vi "_Save All Tables.vi"(4 "error in (no error)":errorcluster, 5 "FilePath(My Table.tbl)":string="My Tables.tbl", 7 "SaveOption (Temporary File)":T1=enum."Temporary File") -> (0 "error out":errorcluster, 1 "Path":path)   [LabVIEW 2015]
uses:
  Type/_SaveOption.ctl
  Type/_RT Command.ctl
  Type/_RT Configuration 2.ctl
  <vilib>/Utility/config.llb/Read Key (String).vi
  Configuration/_Global Configuration.vi
  <vilib>/Utility/config.llb/NI_LVConfig.lvlib
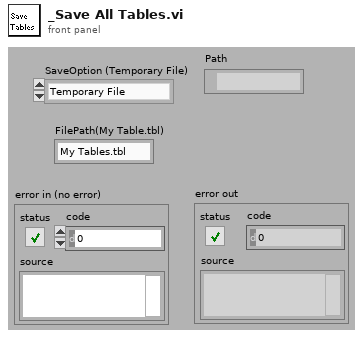
[diagram p1: front panel]
types:
  T1 = typedef "_SaveOption.ctl" = enum16{"Use Dialog", "Temporary File", "My Tables", "Full Path"}
  T2 = typedef "_RT Configuration 2.ctl" = cluster{"Name":string, "Ch#":u8, "Min":dbl, "Max":dbl, "Def+":dbl, "Def-":dbl, "Offset":dbl, "Slope":dbl, "Type":u8, "Description":string, "SettleT":dbl}
  T3 = typedef "_RT Command.ctl" = enum16{"Start", "StartActualRun", "Stop", "Runtime Update", "Get Data", "Get Info", "Get Status", "Get Param", "Get Config", "Get Table", "Read ADC", "Set Oscillator", "Update Config", "Update Table", "Set All Pol", "Set Pol and DC", "Set Max Mass", "Toggle RP", "Toggle EL", "Set PIC", "Initialize Turbo", "Send Turbo Comm", "Close Turbo", "P1", "P2", "P3", "Send Serial", "Set LC Out", "Get LC In", "Read VAC", "Test Table", "Toggle Power", "Get Startup", "Set Startup", "Get ADC Table", "Set ADC Table", "Get Brief Status", "Get Detail Status", "Auxiliary Update", "Set CC Logics", "Set CC Input Logics", "Ignore Error"}
  T4 = enum32{"existing file", "new file", "new or existing file", "existing dir", "new dir", "new or existing dir", "existing file (use LLBs)", "new file (use LLBs)", "new or existing file (use LLBs)", "new or existing file or directory (use LLBs)"}
  T5 = typedef "NI_LVConfig.lvlib/Config Data RefNum.ctl" = refnum<k1>
  T6 = enum16{"open", "replace", "create", "open or create", "replace or create", "replace or create with confirmation"}
  T7 = typedef "_RT Instrument 2.ctl" = cluster{"Table":T2[], "Instrument":string[]}
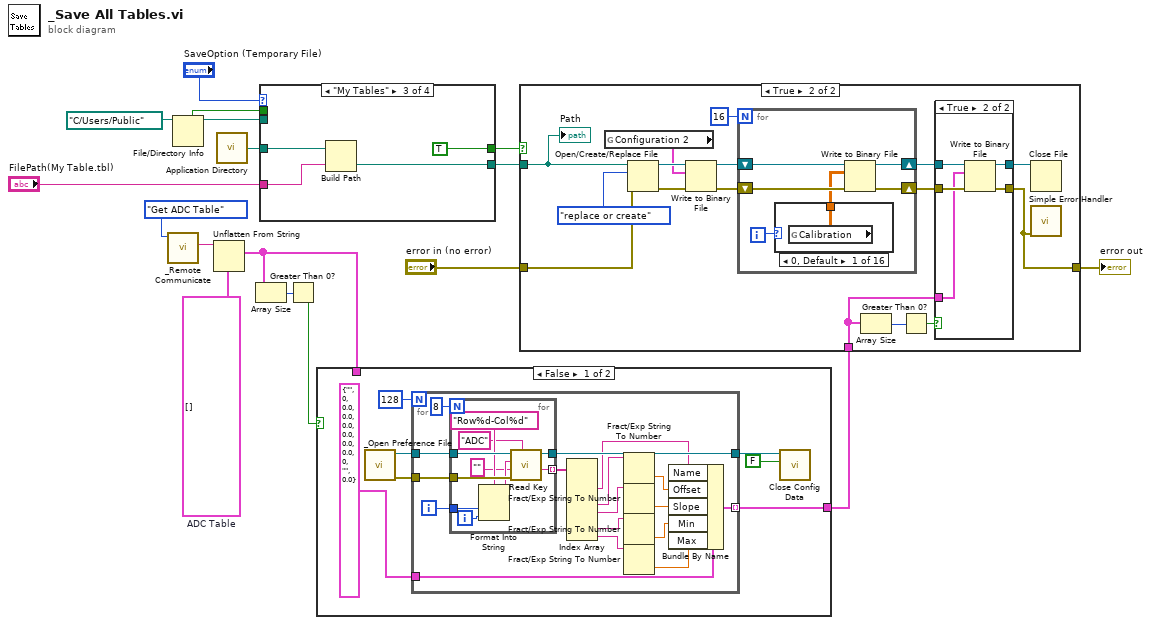
[diagram p0: block diagram]
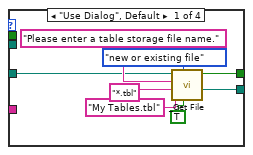
[diagram p3: hidden frame]
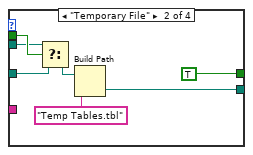
[diagram p4: hidden frame]
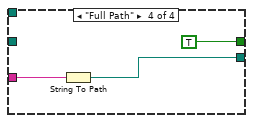
[diagram p5: hidden frame]
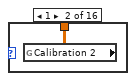
[diagram p8: hidden frame]
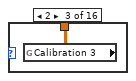
[diagram p9: hidden frame]
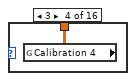
[diagram p10: hidden frame]
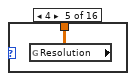
[diagram p11: hidden frame]
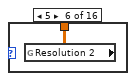
[diagram p12: hidden frame]
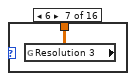
[diagram p13: hidden frame]
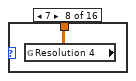
[diagram p14: hidden frame]
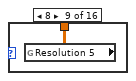
[diagram p15: hidden frame]
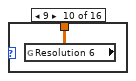
[diagram p16: hidden frame]
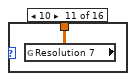
[diagram p17: hidden frame]
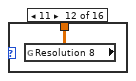
[diagram p18: hidden frame]
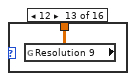
[diagram p19: hidden frame]
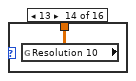
[diagram p20: hidden frame]
diagram:
  w11 = T2[] []  # ADC Table
  n1 = call "_Remote Communicate.vi"("Command"=_RT_Command."Get ADC Table") -> ("Info"=w13:string)  [unwired: 5 in, 3 out]
  n2 = File/Directory Info(path=path "C:/Users/Public" ("stripped path")) -> (path out=w5:path, directory=w6:bool)  [unwired: 1 in, 5 out]
  n3 = Unflatten From String(type=w11, binary string=w13) -> (value=w9:T2[])  [unwired: 1 in, 4 out]
  n4 = call <vilib>:"Application Directory.vi"() -> ("Application Directory"=w1:path)
  n5 = Array Size(array=w9) -> (size(s)=w14:i32)
  n6 = case shown="\"My Tables\"" "SaveOption (Temporary File)" {
    tunnel: w1 -> [w21 w28 w36 _]
    tunnel: [w20 w31 w35 w37] -> w17
    tunnel: [w18 TRUE TRUE TRUE] -> w16
    tunnel: w6 -> [_ w29 _ _]
    tunnel: w5 -> [_ w27 _ _]
    tunnel: "FilePath(My Table.tbl)" -> [_ _ w33 w38]
    frame "Use Dialog", Default {
      n7 = call "_Get File.vi"("For Write (T)"=TRUE, "select mode (new or existing)"=T4."new or existing file", "default name"="My Tables.tbl", "extension (isd)"="*.tbl" ("pattern (all files)"), "prompt"="Please enter a table storage file name.", "Start Path"=w21) -> ("Seleted File"=w20:path, "Succeeded"=w18:bool)  [unwired: 2 out]
    }
    frame "Temporary File" {
      n8 = Select(t=w27, s=w29, f=w28) -> (s? t:f=w26:path)
      n9 = Build Path(base path=w26, name or relative path="Temp Tables.tbl") -> (appended path=w31:path)
    }
    frame "My Tables" {
      n10 = Build Path(base path=w36, name or relative path=w33) -> (appended path=w35:path)
    }
    frame "Full Path" {
      n11 = String To Path(string=w38) -> (path=w37:path)
    }
  }
  n12 = Greater Than 0?(x=w14) -> (x > 0?=w10:bool)
  n13 = case shown="False" w10 {
    tunnel: [w40 w74] -> w8
    tunnel: w9 -> [_ w74]
    frame False {
      n14 = call "_Open Preference File.vi"() -> ("error"=w46:errorcluster, "refnum"=w45:T5)  [unwired: 2 in, 4 out]
      n15 = for {
        N: 128 -> [_]
        tunnel: w45 -> [w63]
        tunnel: w46 -> [w62]
        tunnel: [w60] -> w42
        tunnel: T2 {"Name"="", "Ch#"=0, "Min"=0.0, "Max"=0.0, "Def+"=0.0, "Def-"=0.0, "Offset"=0.0, "Slope"=0.0, "Type"=0, "Description"="", "SettleT"=0.0} ("Configuration") -> [w48]
        tunnel: [w47] -> w40 mode=indexing
        i -> [w59]
        n16 = for {
          N: 8 -> [_]
          tunnel: w63 -> [w73]
          tunnel: w62 -> [w72]
          tunnel: [w71] -> w60
          tunnel: w59 -> [w69]
          tunnel: [w66] -> w54 mode=indexing
          i -> [w70]
          n17 = Format Into String(format string="Row%d-Col%d" ("section"), w69, w70) -> (resulting string=w67:string)  [unwired: 2 in, 1 out]
          n18 = call-poly <vilib>:"Read Key.vi"("section"="ADC", "error in (no error)"=w72, "default value"="", "key"=w67, "refnum"=w73) -> ("value"=w66:string, "refnum out"=w71:T5)  [unwired: 1 in, 4 out]
        }
        n19 = Index Array(array=w54) -> (element #2=w53:string, element #4=w55:string, element #5=w56:string, element #7=w57:string, element #8=w58:string)  [unwired: 8 in, 3 out]
        n20 = Fract/Exp String To Number(string=w55) -> (number=w49:dbl)  [unwired: 4 out]
        n21 = Fract/Exp String To Number(string=w56) -> (number=w50:dbl)  [unwired: 4 out]
        n22 = Fract/Exp String To Number(string=w57) -> (number=w51:dbl)  [unwired: 4 out]
        n23 = Fract/Exp String To Number(string=w58) -> (number=w52:dbl)  [unwired: 4 out]
        n24 = Bundle By Name(cluster=w48, "Name"=w53, "Offset"=w49, "Slope"=w50, "Min"=w51, "Max"=w52) -> (w47:T2)
      }
      n25 = call <vilib>:"Close Config Data.vi"("write file if changed (T)"=FALSE ("write configuration file? (T)"), "refnum"=w42) -> ()  [unwired: 1 in, 9 out]
    }
    frame True {
    }
  }
  n26 = case shown="True" w16 {
    tunnel: w17 -> [_ w79]
    tunnel: w8 -> [_ w80]
    tunnel: "error in (no error)" -> [w75 w78]
    tunnel: [w75 w77] -> w3
    frame False {
    }
    frame True {
      n27 = global read "_Global Configuration.vi" "Configuration 2"() -> (w89:T7)
      n28 = Open/Create/Replace File(file path (use dialog)=w79, error in=w78, operation (0:open)=T6."replace or create") -> (refnum out=w91:refnum<file>, error out=w90:errorcluster)  [unwired: 3 in, 1 out]
      n29 = Write to Binary File(file (use dialog)=w91, data=w89, error in=w90) -> (refnum out=w87:refnum<file>, error out=w88:errorcluster)  [unwired: 4 out]
      n30 = for {
        N: 16 -> [_]
        shift-right: [w99] -> w82
        shift-left: w88 -> [w102]
        shift-right: [w100] -> w83
        shift-left: w87 -> [w103]
        i -> [w104]
        n31 = case shown="0, Default" w104 {
          tunnel: [w105 w106 w107 w108 w109 w110 w111 w112 w113 w114 w115 w116 w117 w118 w119 w120] -> w101
          frame 0, Default {
            n32 = global read "_Global Configuration.vi" "Calibration"() -> (w105:dbl[][])
          }
          frame 1 {
            n33 = global read "_Global Configuration.vi" "Calibration 2"() -> (w106:dbl[][])
          }
          frame 2 {
            n34 = global read "_Global Configuration.vi" "Calibration 3"() -> (w107:dbl[][])
          }
          frame 3 {
            n35 = global read "_Global Configuration.vi" "Calibration 4"() -> (w108:dbl[][])
          }
          frame 4 {
            n36 = global read "_Global Configuration.vi" "Resolution"() -> (w109:dbl[][])
          }
          frame 5 {
            n37 = global read "_Global Configuration.vi" "Resolution 2"() -> (w110:dbl[][])
          }
          frame 6 {
            n38 = global read "_Global Configuration.vi" "Resolution 3"() -> (w111:dbl[][])
          }
          frame 7 {
            n39 = global read "_Global Configuration.vi" "Resolution 4"() -> (w112:dbl[][])
          }
          frame 8 {
            n40 = global read "_Global Configuration.vi" "Resolution 5"() -> (w113:dbl[][])
          }
          frame 9 {
            n41 = global read "_Global Configuration.vi" "Resolution 6"() -> (w114:dbl[][])
          }
          frame 10 {
            n42 = global read "_Global Configuration.vi" "Resolution 7"() -> (w115:dbl[][])
          }
          frame 11 {
            n43 = global read "_Global Configuration.vi" "Resolution 8"() -> (w116:dbl[][])
          }
          frame 12 {
            n44 = global read "_Global Configuration.vi" "Resolution 9"() -> (w117:dbl[][])
          }
          frame 13 {
            n45 = global read "_Global Configuration.vi" "Resolution 10"() -> (w118:dbl[][])
          }
          frame 14 {
            n46 = global read "_Global Configuration.vi" "Resolution 11"() -> (w119:dbl[][])
          }
          frame 15 {
            n47 = global read "_Global Configuration.vi" "Resolution 12"() -> (w120:dbl[][])
          }
        }
        n48 = Write to Binary File(file (use dialog)=w103, data=w101, error in=w102) -> (refnum out=w100:refnum<file>, error out=w99:errorcluster)  [unwired: 4 out]
      }
      n49 = Array Size(array=w80) -> (size(s)=w85:i32)
      n50 = Greater Than 0?(x=w85) -> (x > 0?=w84:bool)
      n51 = case shown="True" w84 {
        tunnel: w80 -> [_ w96]
        tunnel: w83 -> [w93 w98]
        tunnel: w82 -> [w92 w97]
        tunnel: [w93 w95] -> w81
        tunnel: [w92 w94] -> w77
        frame False {
        }
        frame True {
          n52 = Write to Binary File(file (use dialog)=w98, data=w96, error in=w97) -> (refnum out=w95:refnum<file>, error out=w94:errorcluster)  [unwired: 4 out]
        }
      }
      n53 = Close File(refnum=w81) -> ()  [unwired: 1 in, 2 out]
      n54 = call <vilib>:"Simple Error Handler.vi"("error in (no error)"=w77) -> ()  [unwired: 1 in, 8 out]
      "Path" <- w79
    }
  }
  "error out" <- w3
